vi "Read Tree Menu Structure.vi"(4 "Error In":errorcluster, 6 "Menu Context":T1, 7 "Config Data_DB_ADO in":refnum<class "Config Data_DB_ADO.lvclass">) -> (0 "Error Out":errorcluster, 2 "Tree Menu Structure":T2[](array[typedef]), 3 "Config Data_DB_ADO out":refnum<class "Config Data_DB_ADO.lvclass">)   [LabVIEW 2020, in "Config Data.lvlib" / "Config Data_DB_ADO.lvclass"]
uses:
  Config Data_DB_ADO.lvclass
  C:/Users/Fred Guo/Desktop/Release 19/_libraries/Config Data/DB/Config Data_DB.lvclass
  typedefs/Tree Menu Entry.ctl
  typedefs/Menu Context Selections.ctl
  toolbox/ADO Database Drivers/ADO Database Drivers.lvlib
  Config Data_DB.lvclass
  Config Data.lvclass
panel:
  # "`"
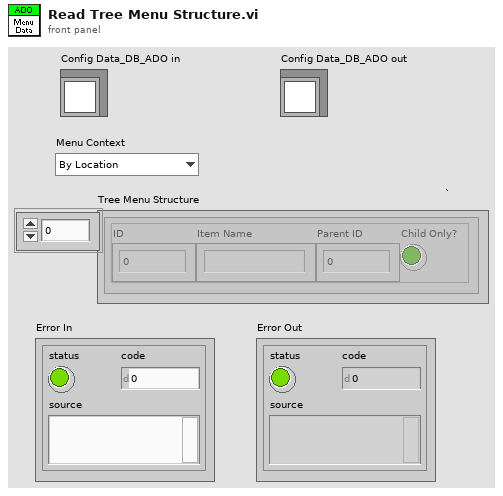
[diagram p1: front panel]
types:
  T1 = typedef "Config Data.lvlib/Config Data.lvclass/Menu Context Selections.ctl" = enum16{"By Location", "By Function"}
  T2 = typedef "Config Data.lvlib/Config Data.lvclass/Tree Menu Entry.ctl" = cluster{"ID":i32, "Item Name":string, "Parent ID":i32, "Child Only?":bool}
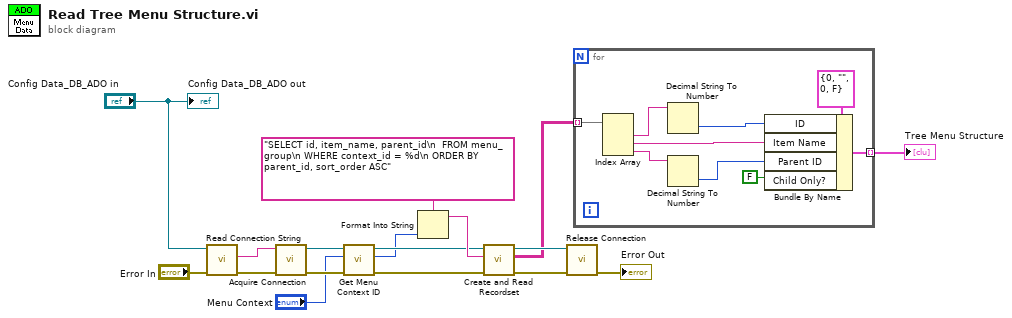
[diagram p0: block diagram]
diagram:
  n1 = call "Read Connection String.vi"("Error In"="Error In", "DB In"="Config Data_DB_ADO in") -> ("Error Out"=w15:errorcluster, "Connection String"=w16:string)  [unwired: 3 in, 1 out]
  n2 = call "Acquire Connection.vi"("error in (no error)"=w15, "Connection String"=w16) -> ("error out"=w5:errorcluster, "Connection"=w6:refnum<k7>)  [unwired: 3 in, 1 out]
  n3 = call "Get Menu Context ID.vi"("error in (no error)"=w5, "Menu Context"="Menu Context", "Connection In"=w6) -> ("error out"=w3:errorcluster, "context_id"=w2:i32, "Connection Out"=w4:refnum<k7>)  [unwired: 2 in]
  n4 = Format Into String(format string="SELECT id, item_name, parent_id\n  FROM menu_group\n WHERE context_id = %d\n ORDER BY parent_id, sort_order ASC", w2) -> (resulting string=w17:string)  [unwired: 2 in, 1 out]
  n5 = call "Create and Read Recordset.vi"("error in (no error)"=w3, "Source"=w17, "Connection In"=w4) -> ("error out"=w10:errorcluster, "DB Data"=w9:string[][], "Connection Out"=w11:refnum<k7>)  [unwired: 2 in, 2 out]
  n6 = call "Release Connection.vi"("error in"=w10, "Connection"=w11) -> ("error out"=→"Error Out":errorcluster)  [unwired: 5 in]
  n7 = for {
    tunnel: w9 -> [w22] mode=indexing
    tunnel: [w18] -> w7 mode=indexing
    n8 = Index Array(array=w22) -> (element #1=w19:string, element #2=w21:string, element #3=w20:string)  [unwired: 3 in]
    n9 = Decimal String To Number(string=w19) -> (number=w25:i32)  [unwired: 2 in, 1 out]
    n10 = Decimal String To Number(string=w20) -> (number=w23:i32)  [unwired: 2 in, 1 out]
    n11 = Bundle By Name(cluster=T2 {"ID"=0, "Item Name"="", "Parent ID"=0, "Child Only?"=FALSE}, "ID"=w25, "Item Name"=w21, "Parent ID"=w23, "Child Only?"=FALSE) -> (w18:T2)
  }
  "Tree Menu Structure" <- w7
  "Config Data_DB_ADO out" <- "Config Data_DB_ADO in"
